vi "Transfer Group.Create.vi"(4 "engine offset":u64, 5 "Debug Flags":refnum<class "Debug Flags.lvclass">, 6 "transceiver id":i32, 7 "framework id":i32, 8 "error in (no error)":errorcluster, 9 "Direction":T1, 10 "Timing":refnum<class "Timing.lvclass">, 11 "Transfers":refnum<class "Transfer.lvclass">[](array[class])) -> (0 "error out":errorcluster, 3 "Transfer Group out":refnum<class "Transfer Group.lvclass">)   [LabVIEW 2017, in "DSF Core.lvlib" / "Transfer Group.lvclass"]
uses:
  Transfer Group.lvclass
  Transfer.lvclass
  Timing/Timing.lvclass
  DSF Configuration API/Public/Controls/DSF Direction.ctl
  Debug/Debug Flags/Debug Flags.lvclass
  Transfer Group.lvclass/Transfer Group.ctl
  DSF Core.lvlib
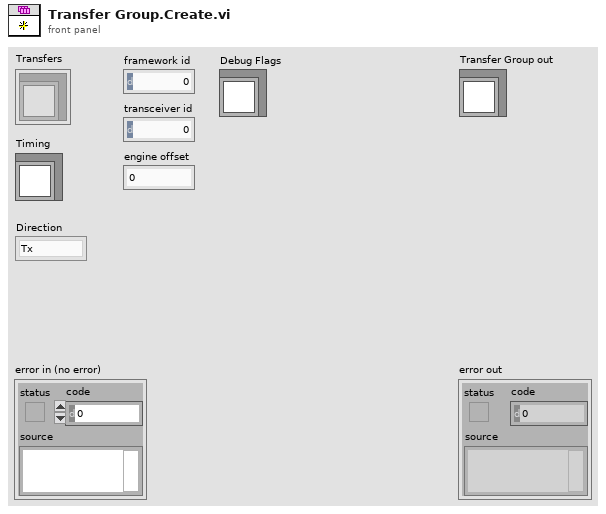
[diagram p1: front panel]
types:
  T1 = typedef "DSF Core.lvlib/DSF Direction.ctl" = enum8{"Tx", "Rx"}
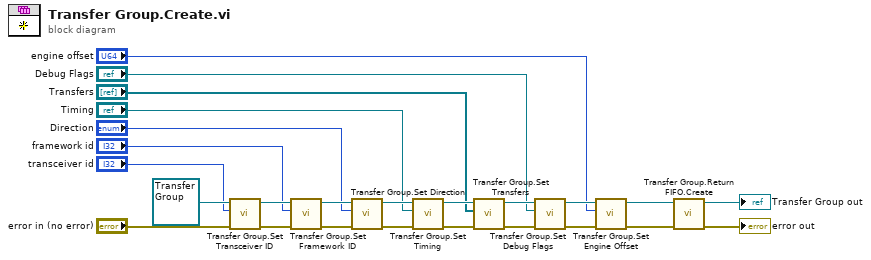
[diagram p0: block diagram]
diagram:
  n1 = call "Transfer Group.Set Transceiver ID.vi"("transceiver id"="transceiver id", "Transfer Group in"=refnum<class "Transfer Group.lvclass"> refnum ("Transfer Group type")) -> ("Transfer Group out"=w7:refnum<class "Transfer Group.lvclass">)  [unwired: 9 in]
  n2 = call "Transfer Group.Set Framework ID.vi"("framework id"="framework id", "Transfer Group in"=w7) -> ("Transfer Group out"=w18:refnum<class "Transfer Group.lvclass">)  [unwired: 9 in]
  n3 = call "Transfer Group.Set Direction.vi"("Direction"="Direction", "Transfer Group in"=w18) -> ("Transfer Group out"=w17:refnum<class "Transfer Group.lvclass">)  [unwired: 9 in]
  n4 = call "Transfer Group.Set Timing.vi"("Timing"="Timing", "Transfer Group in"=w17) -> ("Transfer Group out"=w16:refnum<class "Transfer Group.lvclass">)  [unwired: 9 in]
  n5 = call "Transfer Group.Set Transfers.vi"("Transfers"="Transfers", "Transfer Group in"=w16) -> ("Transfer Group out"=w9:refnum<class "Transfer Group.lvclass">)  [unwired: 9 in]
  n6 = call "Transfer Group.Set Debug Flags.vi"("Debug Flags"="Debug Flags", "Transfer Group in"=w9) -> ("Transfer Group out"=w3:refnum<class "Transfer Group.lvclass">)  [unwired: 9 in]
  n7 = call "Transfer Group.Set Engine Offset.vi"("engine offset"="engine offset", "Transfer Group in"=w3) -> ("Transfer Group out"=w2:refnum<class "Transfer Group.lvclass">)  [unwired: 9 in]
  n8 = call "Transfer Group.Return FIFO.Create.vi"("error in (no error)"="error in (no error)", "Transfer Group in"=w2) -> ("error out"=→"error out":errorcluster, "Transfer Group out"=→"Transfer Group out":refnum<class "Transfer Group.lvclass">)  [unwired: 8 in]
